vi "Power Fit.vi"(0 "Y":dbl[](array[numeric]), 5 "X":dbl[](array[numeric]), 7 "Weight":dbl[](array[numeric]), 9 "tolerance":dbl=0.0001 format="%#_3g", 11 "method":T2 items=["Least Square", "Least Absolute Residual", "Bisquare"], 12 "parameter bounds":T1={"amp min"=-inf, "amp max"=inf, "power min"=-inf, "power max"=inf, "offset min"=0.0, "offset max"=0.0}) -> (4 "Best Power Fit":dbl[](array[numeric]), 6 "amplitude":dbl, 8 "power":dbl, 10 "offset":dbl, 14 "residue":dbl, 15 "error":i32)   [LabVIEW 2017, in "NI_AALPro.lvlib"]
doc: "Returns the power fit of a data set (<B>X</B>, <B>Y</B>) using the Least Square, Least Absolute Residual, or Bisquare method."
uses:
  <vilib>/Analysis/NI_AALPro.lvlib
  <vilib>/Analysis/6fits.llb/Curve Fitting Criteria.ctl
  <resource>/lvanlys.dll
panel:
  # "Constrained Power Fit"
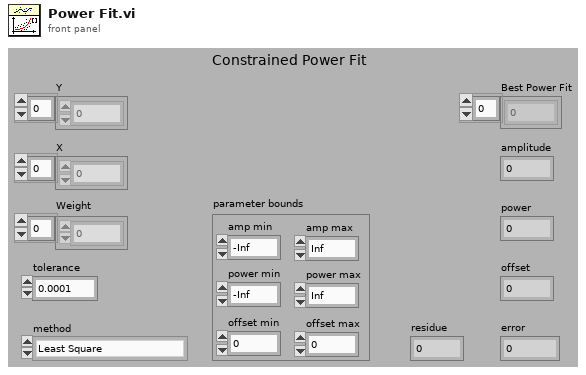
[diagram p1: front panel]
types:
  T1 = cluster{"amp min":dbl, "amp max":dbl, "power min":dbl, "power max":dbl, "offset min":dbl, "offset max":dbl}
  T2 = typedef "NI_AALPro.lvlib/Curve Fitting Criteria.ctl" = u16
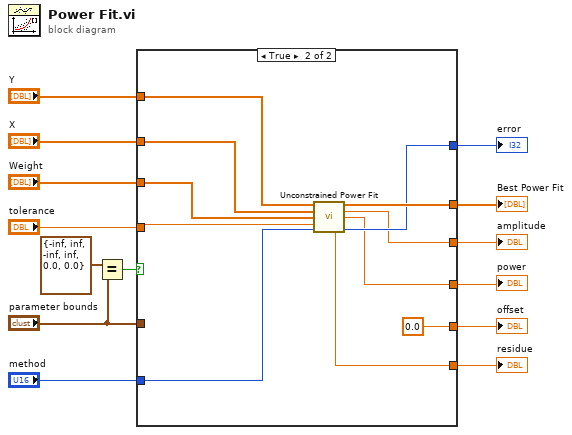
[diagram p0: block diagram]
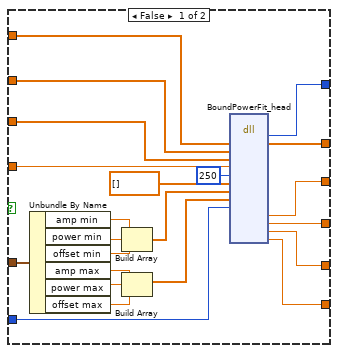
[diagram p2: hidden frame]
diagram:
  n1 = Equal?(x=T1 {"amp min"=-inf, "amp max"=inf, "power min"=-inf, "power max"=inf, "offset min"=0.0, "offset max"=0.0} ("parameter bounds 2"), y="parameter bounds") -> (x = y?=w1:bool)
  n2 = case shown="True" w1 {
    tunnel: "Y" -> [w35 w47]
    tunnel: "X" -> [w34 w40]
    tunnel: "Weight" -> [w33 w39]
    tunnel: "tolerance" -> [w32 w38]
    tunnel: "method" -> [w30 w37]
    tunnel: [w29 w45] -> w9
    tunnel: [w28 w46] -> w8
    tunnel: [w27 w44] -> w7
    tunnel: [w26 w43] -> w6
    tunnel: [w25 w42] -> w5
    tunnel: "parameter bounds" -> [w18 _]
    tunnel: [w15 0.0 ("offset")] -> w4
    frame False {
      n3 = Unbundle By Name(w18) -> ("amp min"=w24:dbl, "power min"=w23:dbl, "offset min"=w22:dbl, "amp max"=w21:dbl, "power max"=w20:dbl, "offset max"=w19:dbl)
      n4 = Build Array(w24, w23, w22) -> (w16:dbl[])
      n5 = Build Array(w21, w20, w19) -> (w17:dbl[])
      n6 = dll-call lib="e:/builds/penguin/labview/branches/2017/dev/dist/resource/lvanlys.*" fn="BoundPowerFit_head"("y"=w35, "x"=w34, "weight"=w33, "tolerance"=w32, "maxIter"=250, "intial coef"=dbl[] [] ("initial coefficients"), "minBound"=w16, "maxBound"=w17, "algorithm"=w30) -> ("return type"=w29:i32, "y"=w28:dbl[], "amp"=w27:dbl, "power"=w26:dbl, "offset"=w15:dbl, "residue"=w25:dbl)  [unwired: 9 in, 8 out]
    }
    frame True {
      n7 = call <vilib>:"Unconstrained Power Fit.vi"("Y"=w47, "X"=w40, "Weight"=w39, "tolerance"=w38, "method"=w37) -> ("Best Power Fit"=w46:dbl[], "amplitude"=w44:dbl, "power"=w43:dbl, "residue"=w42:dbl, "error"=w45:i32)  [unwired: 6 out]
    }
  }
  "power" <- w6
  "amplitude" <- w7
  "Best Power Fit" <- w8
  "offset" <- w4
  "error" <- w9
  "residue" <- w5
